vi "Robot Main.vi"() -> ()   [LabVIEW 2019]
doc: "This VI implements the framework and scheduler for your robotics program. It should not be necessary to modify the framework. You are expected to add your code to the VIs called from Robot Main - the ones located in the Team Code folder within the project."
uses:
  <vilib>/Rock Robotics/WPI/Camera/WPI_CameraImageSize.ctl
  <vilib>/Rock Robotics/SystemInterfaces/i2clib/i2c_bus.ctl
  Robot Global Data.vi
panel:
  in  "Finish 3":bool
  out "error out 2":errorcluster
  out "Proximity 2":u16(graph)
  out "Matched Color Name 2":string
  out "Match Confidence 2":dbl
  out "Color 2":u32(colorbox)
  out "Measured Color 2":cluster{"R":dbl, "G":dbl, "B":dbl}
  in  "I2C Bus 2":T1
  in  "Blue Calibration":cluster{"R":dbl, "G":dbl, "B":dbl}={"R"=0.143, "G"=0.427, "B"=0.429}
  in  "Green Calibration":cluster{"R":dbl, "G":dbl, "B":dbl}={"R"=0.197, "G"=0.561, "B"=0.24}
  in  "Red Calibration":cluster{"R":dbl, "G":dbl, "B":dbl}={"R"=0.561, "G"=0.323, "B"=0.114}
  in  "Yellow Calibration":cluster{"R":dbl, "G":dbl, "B":dbl}={"R"=0.361, "G"=0.524, "B"=0.113}
  in  "Image Size":T2=enum."320x240"
  in  "Enable Vision":bool
  in  "Finish":bool
  # "Target Calibration (Latched at the start)"
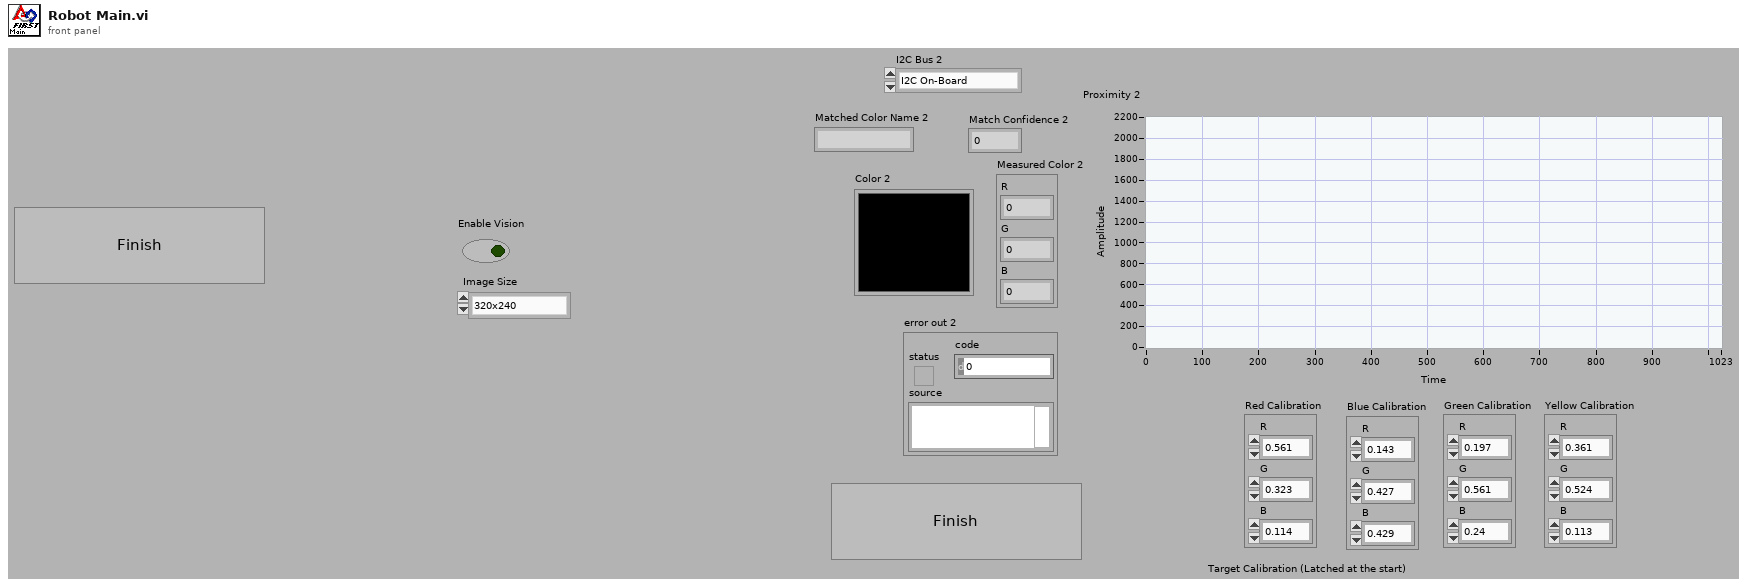
[diagram p1: front panel]
types:
  T1 = typedef "i2c_bus.ctl" = enum16{"I2C On-Board", "I2C MXP", "Invalid"}
  T2 = typedef "WPI_CameraImageSize.ctl" = enum16{"640x480", "320x240", "160x120", "Custom"}
  T3 = typedef "Color Sensor V3 DevRef.ctl" = cluster{"I2CDevRef":T4}
  T4 = typedef "WPI_I2CDevRef.ctl" = cluster{"DevStatus":errorcluster, "Device Address":u8, "Handle":i32, "I2C Bus":T1}
  T5 = typedef "WPI_DriverStationMatch Info.ctl" = cluster{"Autonomous Elapsed Seconds":dbl, "TeleOp Elapsed Seconds":dbl, "Disabled Elapsed Seconds":dbl, "Visited Autonomous":bool, "Visited TeleOp":bool, "Visited Disabled":bool, "Autonomous Settings":cluster{"Autonomous Style":enum16{"Iterative", "Independent"}, "VI Refnum":refnum<vi>}}
  T6 = typedef "WPI_DriverStationDerivedRobotMode.ctl" = enum16{"Init", "Execute", "Stop"}
  T7 = typedef "WPI_DriverStationRobotMode2.ctl" = enum16{"Autonomous Disabled", "Autonomous Enabled", "Teleop Disabled", "Teleop Enabled", "Disconnected", "Finish", "Test Disabled", "Test Enabled", "Emergency Stopped"}
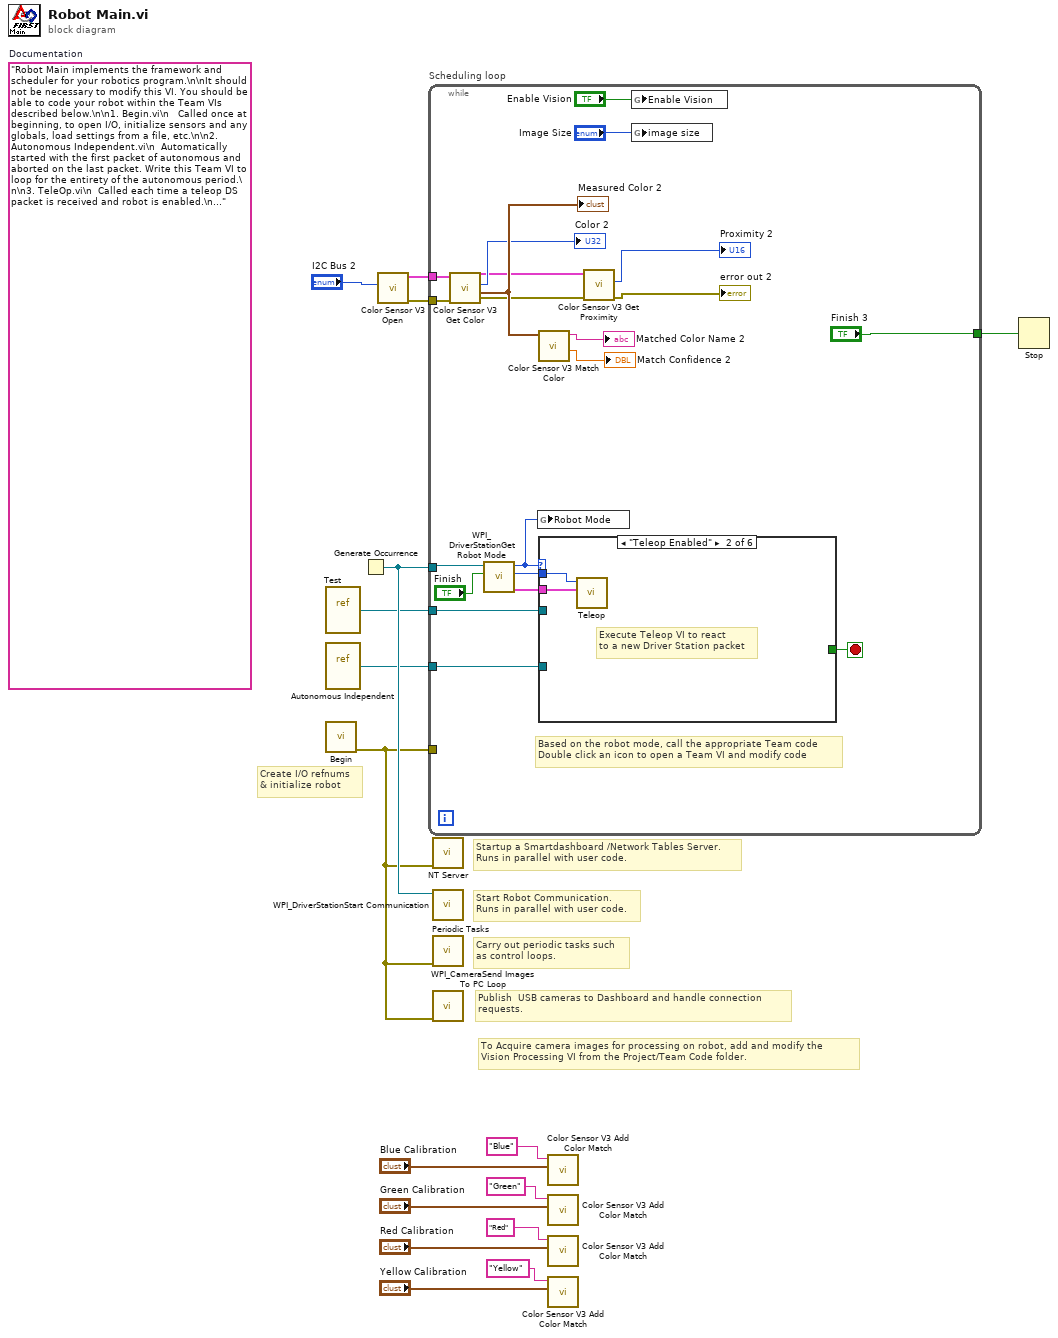
[diagram p0: block diagram]
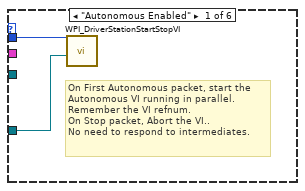
[diagram p2: hidden frame]
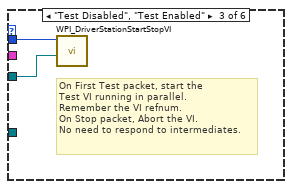
[diagram p3: hidden frame]
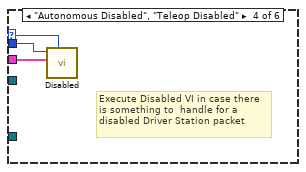
[diagram p4: hidden frame]
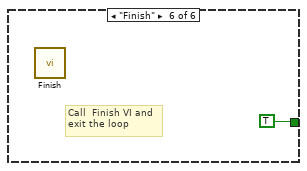
[diagram p6: hidden frame]
diagram:
  (unwired) "Robot Main implements the framework and scheduler for your robotics program.\n\nIt should not be necessary to modify this VI. You should be able to code your robot within the Team VIs described below.\n\n1. Begin.vi\n   Called once at beginning, to open I/O, initialize sensors and any globals, load settings from a file, etc.\n\n2. Autonomous Independent.vi\n  Automatically started with the first packet of autonomous and aborted on the last packet. Write this Team VI to loop for the entirety of the autonomous period.\n\n3. TeleOp.vi\n  Called each time a teleop DS packet is received and robot is enabled.\n\n4. Disabled.vi\n  Called each time a packet is received and the robot is disabled.\n\n5. Test.vi\n  Called Automatically started with the first test packet and aborted on the last. Modify this VI to carry out robot and sensor validation tests.\n\n6. Vision Processing.vi\n  A parallel loop that acquires and processes camera images. Drag from the project/Team Code if you wish to use this.\n\n7. PeriodicTasks.vi\n  Parallel loops running at user-defined rates.\n\n8. Finish.vi\n  Called before exiting, so you can save data, clean up I/O, etc.\n"  # Documentation
  # "Publish  USB cameras to Dashboard and handle connection\nrequests."
  # "Startup a Smartdashboard /Network Tables Server.\nRuns in parallel with user code."
  # "Carry out periodic tasks such\nas control loops."
  # "To Acquire camera images for processing on robot, add and modify the\nVision Processing VI from the Project/Team Code folder."
  # "Create I/O refnums\n& initialize robot"
  # "Start Robot Communication.\nRuns in parallel with user code."
  n1 = vi-ref "Test.vi"() -> (w14:refnum<vi>)
  n2 = vi-ref "Autonomous Independent.vi"() -> (w15:refnum<vi>)
  n3 = call "Begin.vi"() -> ("error out"=w13:errorcluster)  [unwired: 2 in, 9 out]
  n4 = Generate Occurrence() -> (w16:refnum<k4>)
  n5 = call <vilib>:"Color Sensor V3 Open.vi"("I2C Bus"="I2C Bus 2") -> ("error out"=w2:errorcluster, "ColorSensorDevRef"=w3:T3)  [unwired: 9 in]
  n6 = while "Scheduling loop" {
    tunnel: w16 -> [w36]
    tunnel: w13 -> [_]
    tunnel: w15 -> [w31]
    tunnel: w14 -> [w29]
    tunnel: w3 -> [w27]
    tunnel: w2 -> [w26]
    tunnel: ["Finish 3"] -> w1
    stop <- w33 stop-if-true
    # "Based on the robot mode, call the appropriate Team code\nDouble click an icon to open a Team VI and modify code"
    n7 = call <vilib>:"Color Sensor V3 Get Color.vi"("error in (no error)"=w26, "ColorSensorDevRef"=w27) -> ("error out"=w20:errorcluster, "Normalized Color"=w25:cluster{"R":dbl, "G":dbl, "B":dbl}, "Color"=→"Color 2":u32, "ColorSensorDevRef out"=w21:T3)  [unwired: 6 in]
    "Measured Color 2" <- w25
    n8 = call <vilib>:"WPI_DriverStationGet Robot Mode.vi"("Finish"="Finish", "DS Occurrence"=w36) -> ("Match Info out"=w34:T5, "Call Context"=w37:T6, "Robot Mode"=w28:T7)  [unwired: 7 out]
    n9 = global write "Robot Global Data.vi" "Robot Mode"(w28) -> ()
    n10 = call <vilib>:"Color Sensor V3 Match Color.vi"("Measured Color"=w25) -> ("Confidence"=→"Match Confidence 2":dbl, "Matched Color Name"=→"Matched Color Name 2":string)  [unwired: 8 in, 1 out]
    n11 = case shown="\"Teleop Enabled\"" w28 {
      selector: w28 -> [_ _ _ w44 _ _]
      tunnel: w37 -> [w39 w41 w43 w46 _ _]
      tunnel: w34 -> [_ w40 _ w45 _ _]
      tunnel: [_ _ _ _ _ TRUE] -> w33
      tunnel: w31 -> [w38 _ _ _ _ _]
      tunnel: w29 -> [_ _ w42 _ _ _]
      frame "Autonomous Enabled" {
        # "On First Autonomous packet, start the\nAutonomous VI running in parallel.\nRemember the VI refnum.\nOn Stop packet, Abort the VI..\nNo need to respond to intermediates."
        n12 = call <vilib>:"WPI_DriverStationStartStopVI.vi"("VI in"=w38, "Call Context"=w39) -> ()  [unwired: 10 in]
      }
      frame "Teleop Enabled" {
        # "Execute Teleop VI to react\nto a new Driver Station packet"
        n13 = call "Teleop.vi"("Match Info"=w40, "Call Context"=w41) -> ()  [unwired: 1 in, 9 out]
      }
      frame "Test Disabled", "Test Enabled" {
        # "On First Test packet, start the\nTest VI running in parallel.\nRemember the VI refnum.\nOn Stop packet, Abort the VI.\nNo need to respond to intermediates."
        n14 = call <vilib>:"WPI_DriverStationStartStopVI.vi"("VI in"=w42, "Call Context"=w43) -> ()  [unwired: 10 in]
      }
      frame "Autonomous Disabled", "Teleop Disabled" {
        # "Execute Disabled VI in case there\nis something to  handle for a\ndisabled Driver Station packet"
        n15 = call "Disabled.vi"("Robot Mode"=w44, "Match Info"=w45, "Call Context"=w46) -> ()  [unwired: 1 in, 8 out]
      }
      frame "Disconnected", Default {
        # "Driver Station packet didn't arrive.\nPossibly useful for diagnostics"
      }
      frame "Finish" {
        # "Call  Finish VI and\nexit the loop"
        n16 = call "Finish.vi"() -> ()  [unwired: 1 in, 7 out]
      }
    }
    n17 = call <vilib>:"Color Sensor V3 Get Proximity.vi"("error in (no error)"=w20, "ColorSensorDevRef"=w21) -> ("error out"=→"error out 2":errorcluster, "Proximity"=→"Proximity 2":u16)  [unwired: 7 in, 1 out]
    n18 = global write "Robot Global Data.vi" "Enable Vision"("Enable Vision") -> ()
    n19 = global write "Robot Global Data.vi" "image size"("Image Size") -> ()
  }
  n20 = call <vilib>:"NT Server.vi"("error in (no error)"=w13) -> ()  [unwired: 11 in]
  n21 = call <vilib>:"WPI_DriverStationStart Communication.vi"("occurrence"=w16) -> ()  [unwired: 1 in, 10 out]
  n22 = call "Periodic Tasks.vi"("error in"=w13) -> ()  [unwired: 1 in, 10 out]
  n23 = call <vilib>:"WPI_CameraSend Images To PC Loop.vi"("error in (no error)"=w13) -> ()  [unwired: 11 in]
  n24 = call <vilib>:"Color Sensor V3 Add Color Match.vi"("Color"="Blue Calibration", "Name"="Blue") -> ()  [unwired: 10 in]
  n25 = call <vilib>:"Color Sensor V3 Add Color Match.vi"("Color"="Green Calibration", "Name"="Green") -> ()  [unwired: 10 in]
  n26 = call <vilib>:"Color Sensor V3 Add Color Match.vi"("Color"="Red Calibration", "Name"="Red") -> ()  [unwired: 10 in]
  n27 = call <vilib>:"Color Sensor V3 Add Color Match.vi"("Color"="Yellow Calibration", "Name"="Yellow") -> ()  [unwired: 10 in]
  n28 = Stop(stop? (T)=w1) -> ()
